vi "COM Port Detect_Motion.vi"(8 "error in":errorcluster) -> (0 "error out":errorcluster, 2 "Motion Find?":bool, 3 "VISA motion":refnum<visa-resource-name>)   [LabVIEW 2019, in "Allmotion.lvlib"]
uses:
  <vilib>/Instr/_visa.llb/VISA Find Search Mode.ctl
  <vilib>/Instr/_visa.llb/VISA Configure Serial Port (Instr).vi
  Allmotion.lvlib
panel:
  out "find list":string[](array[string])
  out "Description":string[](array[string])
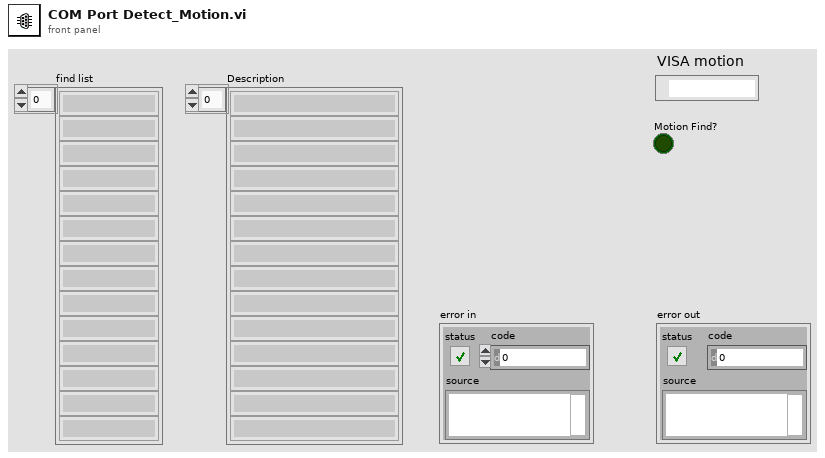
[diagram p1: front panel]
types:
  T1 = typedef "VISA Find Search Mode.ctl" = u32
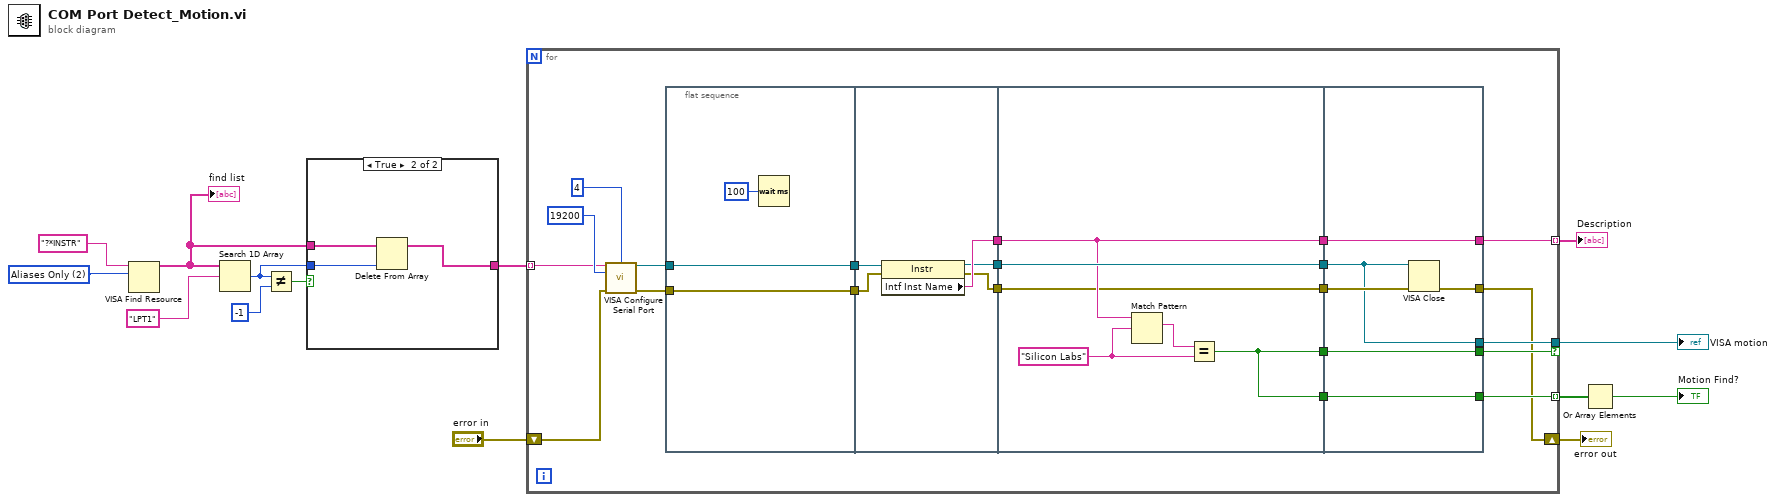
[diagram p0: block diagram]
diagram:
  w13 = T1 2 items=["Canonical Names Only"=0, "Aliases Only"=2, "Include Matching Aliases"=3, "Include All Aliases"=4] ("Search Mode")
  n1 = VISA Find Resource(10:w13, 11:"?*INSTR" ("expression (\"?*\")")) -> (3:w6:string[])  [unwired: 1 in, 2 out]
  "find list" <- w6
  n2 = Search 1D Array(1D array=w6, element="LPT1") -> (index of element=w4:i32)  [unwired: 1 in]
  n3 = Not Equal?(x=w4, y=-1) -> (x != y?=w7:bool)
  n4 = case shown="True" w7 {
    tunnel: w6 -> [w15 w18]
    tunnel: [w15 w16] -> w5
    tunnel: w4 -> [_ w17]
    frame False {
    }
    frame True {
      n5 = Delete From Array(array=w18, index=w17) -> (array with subset deleted=w16:string[])  [unwired: 1 in, 1 out]
    }
  }
  n6 = for {
    tunnel: w5 -> [w21] mode=indexing
    tunnel: [w27] -> w1 if=w25
    tunnel: [w23] -> w12 mode=indexing
    tunnel: [w22] -> w10 mode=indexing
    shift-right: [w20] -> w2
    shift-left: "error in" -> [w19]
    n7 = call-poly "VISA Configure Serial Port"("VISA resource name"=w21, "termination char\n(0xA = '\\n' = LF)"=u8 4 ("termination char\n(0xA = '\\n' = LF)"), "baud rate (9600)"=u32 19200, "error in (no error)"=w19) -> ("VISA resource name out"=w37:refnum<visa-resource-name>, "error out"=w36:errorcluster)  [unwired: 10 in]
    n8 = flat-sequence {
      tunnel: w36 -> [w41]
      tunnel: w37 -> [w42]
      tunnel: [w42] -> w35
      tunnel: [w41] -> w34
      tunnel: w35 -> [w47]
      tunnel: w34 -> [w46]
      tunnel: [w45] -> w33
      tunnel: [w44] -> w31
      tunnel: [w43] -> w28
      tunnel: w33 -> [w52]
      tunnel: [w52] -> w32
      tunnel: w31 -> [w53]
      tunnel: [w53] -> w30
      tunnel: [w49] -> w29
      tunnel: w28 -> [w49]
      tunnel: [w48] -> w26
      tunnel: [w48] -> w24
      tunnel: w32 -> [w55]
      tunnel: w30 -> [w58]
      tunnel: w29 -> [w59]
      tunnel: [w58] -> w27
      tunnel: w26 -> [w57]
      tunnel: [w57] -> w25
      tunnel: w24 -> [w56]
      tunnel: [w56] -> w23
      tunnel: [w55] -> w22
      tunnel: [w54] -> w20
      frame #0 {
        n9 = Wait (ms)(milliseconds to wait=u32 100) -> ()  [unwired: 1 out]
      }
      frame #1 {
        n10 = property class="Instr"(reference=w47, error in=w46) -> (reference out=w44:refnum<visa-resource-name>, error out=w43:errorcluster, "Intf Inst Name"=w45:string)
      }
      frame #2 {
        w50 = "Silicon Labs" ("regular expression")
        n11 = Match Pattern(string=w52, regular expression=w50) -> (match substring=w51:string)  [unwired: 1 in, 3 out]
        n12 = Equal?(x=w51, y=w50) -> (x = y?=w48:bool)
      }
      frame #3 {
        n13 = VISA Close(VISA resource name=w58, error in (no error)=w59) -> (error out=w54:errorcluster)
      }
    }
  }
  "VISA motion" <- w1
  "Description" <- w10
  "error out" <- w2
  n14 = Or Array Elements(Boolean array=w12) -> (logical OR=→"Motion Find?":bool)
